vi "myRIO_BRig_RT__Case_Exp_State_Cue1Pre__v3.vi"(0 "input_dataCurrent":u16[](array[numeric]), 1 "input_dataExp":u16[](array[numeric]), 5 "input_arrTrig":bool[](array[boolean]), 6 "input_spout":enum16{"Left", "Right"}(ring)) -> (9 "output_audioR":bool, 11 "output_audioL":bool, 12 "output_state":T1, 13 "output_CueLed":bool, 14 "output_dataCurrent":u16[](array[numeric]), 16 "output_l1_laserEvent":bool, 17 "output_l1_laserOn":bool, 18 "output_l2_laserEvent":bool, 19 "output_l2_laserOn":bool)   [LabVIEW 2014]
uses:
  myRIO_BRig_RT__Case_Exp_stateList.ctl
panel:
  in  "input_I_lick":bool
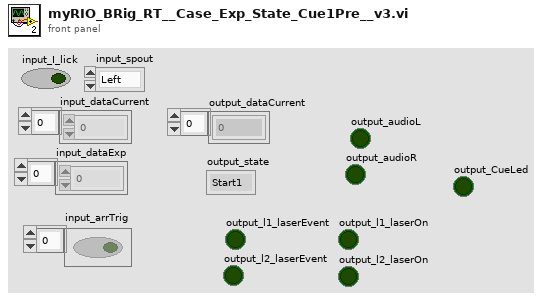
[diagram p1: front panel]
types:
  T1 = typedef "myRIO_BRig_RT__Case_Exp_stateList.ctl" = enum16{"Start1", "Start2", "Start3", "saveSettings1", "saveSettings2", "saveSettings3", "saveSettings4", "saveSettings_LC_ENL_l1", "saveSettings_LC_ENL_l2", "saveSettings_LC_Cue_l1", "saveSettings_LC_Cue_l2", "saveSettings6_LC_l1_Other", "SaveSettings6_LC_l2_Other", "setSettings_Audio", "setSettings_Laser", "initBlock_pre", "initBlock", "initBlock2", "initBlock_post", "initTrial_pre", "initTrial", "initTrial2", "initTrial3", "initTrial4", "initTrial_LC_ENL1", "initTrial_LC_Cue1", "initTrial_LC_Cue1_2", "initTrial_LC_Sel", "initTrial_post", "ENL1_pre", "ENL1", "ENL1_post", "ENL1Penalty_pre", "ENL1Penalty", "ENL2_pre", "ENL2", "ENL2Penalty_pre", "ENL2Penalty", "Cue1_pre", "Cue1", "Cue1_post", "Cue1Penalty_pre", "Cue1Penalty", "Cue2_pre", "Cue2", "Cue2Penalty_pre", "Cue2Penalty", "Selection_pre", "Selection", "Select_post", "SelectReward_pre", "SelectReward", "SelectRewardPost_pre", "SelectRewardPost", "SelectWrong_pre", "SelectWrong", "SelectWrong_post", "SelectTimeout_pre", "SelectTimeout", "SelectTimeout_post", "endTrial_pre", "endTrial1", "endTrial2", "endTrial3", "endTrial_post", "endBlock_pre", "endBlock", "endBlock_post", "endExp", "commConnect", "commUpload_pre", "commUpload_dataBlock", "commUpload_dataCurrent", "commUpload_dataExp", "commUpload_dataLC", "commUpload_dataTrial", "commUpload_post", "saveData_pre", "saveData_dataBlock", "saveData_dataCurrent", "saveData_dataExp", "saveData_dataLC", "saveData_dataTrial", "saveData_post", "empty_endBlock1", "empty_endBlock2", "empty_endTrial1", "empty_endTrial2", "empty_endTrial3", "empty_endTrial4", "empty_endTrial5", "dummyState", "dummyState_endBlock"}
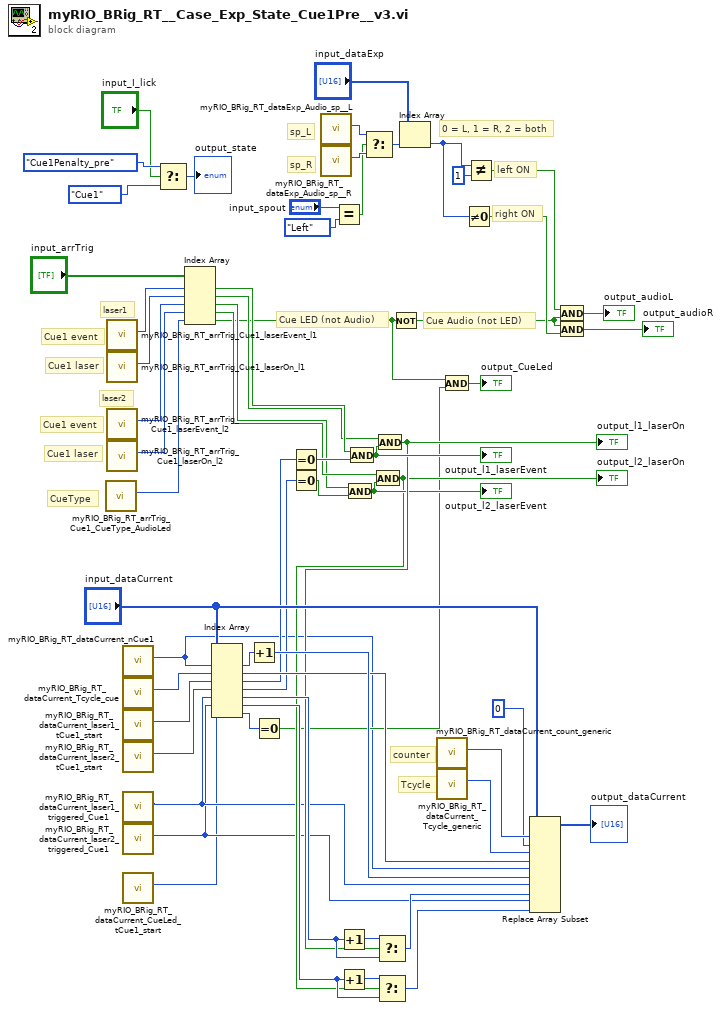
[diagram p0: block diagram]
diagram:
  # "right ON"
  # "left ON"
  # "Cue Audio (not LED)"
  # "Cue LED (not Audio)"
  # "CueType"
  # "0 = L, 1 = R, 2 = both"
  # "sp_R"
  # "sp_L"
  # "Cue1 event"
  # "Cue1 laser"
  # "Cue1 event"
  # "Cue1 laser"
  # "laser2"
  # "laser1"
  # "Tcycle"
  # "counter"
  n1 = call "myRIO_BRig_RT_arrTrig_Cue1_CueType_AudioLed.vi"() -> ("output_arrTrig_Cue1_CueType_AudioLed"=w12:i32)  [unwired: 11 in]
  n2 = call "myRIO_BRig_RT_arrTrig_Cue1_laserEvent_l1.vi"() -> ("output_arrTrig_Cue1_laserEvent_l1"=w25:i32)  [unwired: 11 in]
  n3 = call "myRIO_BRig_RT_arrTrig_Cue1_laserOn_l1.vi"() -> ("output_arrTrig_Cue1_laserOn_l1"=w24:i32)  [unwired: 11 in]
  n4 = call "myRIO_BRig_RT_arrTrig_Cue1_laserEvent_l2.vi"() -> ("output_arrTrig_Cue1_laserEvent_l2"=w23:i32)  [unwired: 11 in]
  n5 = call "myRIO_BRig_RT_arrTrig_Cue1_laserOn_l2.vi"() -> ("output_arrTrig_Cue1_laserOn_l2"=w22:i32)  [unwired: 11 in]
  n6 = call "myRIO_BRig_RT_dataCurrent_nCue1.vi"() -> ("output_nCue1"=w1:i32)  [unwired: 11 in]
  n7 = call "myRIO_BRig_RT_dataCurrent_Tcycle_cue.vi"() -> ("output_Tcycle_cue"=w30:i32)  [unwired: 11 in]
  n8 = call "myRIO_BRig_RT_dataCurrent_laser1_tCue1_start.vi"() -> ("output_laser1_tCue1_start"=w29:i32)  [unwired: 11 in]
  n9 = call "myRIO_BRig_RT_dataCurrent_laser2_tCue1_start.vi"() -> ("output_laser2_tCue1_start"=w28:i32)  [unwired: 11 in]
  n10 = call "myRIO_BRig_RT_dataCurrent_laser1_triggered_Cue1.vi"() -> ("output_laser1_triggered_Cue1"=w27:i32)  [unwired: 11 in]
  n11 = call "myRIO_BRig_RT_dataCurrent_laser2_triggered_Cue1.vi"() -> ("output_laser2_triggered_Cue1"=w26:i32)  [unwired: 11 in]
  n12 = call "myRIO_BRig_RT_dataCurrent_CueLed_tCue1_start.vi"() -> ("output_CueLed_tCue1_start"=w6:i32)  [unwired: 11 in]
  n13 = Select(t=myRIO_BRig_RT__Case_Exp_stateList."Cue1Penalty_pre" ("Enum"), s="input_I_lick", f=myRIO_BRig_RT__Case_Exp_stateList."Cue1" ("Enum")) -> (s? t:f=→"output_state":T1)
  n14 = Index Array(array="input_arrTrig", index #1=w25, index #2=w24, index #3=w23, index #4=w22, index #5=w12) -> (element #1=w40:bool, element #2=w38:bool, element #3=w33:bool, element #4=w34:bool, element #5=w3:bool)
  n15 = Index Array(array="input_dataCurrent", index #1=w1, index #2=w30, index #3=w29, index #4=w28, index #5=w27, index #6=w26, index #7=w6) -> (element #1=w53:u16, element #2=w51:u16, element #3=w50:u16, element #4=w49:u16, element #5=w45:u16, element #6=w44:u16, element #7=w5:u16)
  n16 = Increment(x=w53) -> (x+1=w52:u16)
  n17 = Equal To 0?(x=w5) -> (x = 0?=w4:bool)
  n18 = Equal To 0?(x=w50) -> (x = 0?=w41:bool)
  n19 = Equal To 0?(x=w49) -> (x = 0?=w32:bool)
  n20 = call "myRIO_BRig_RT_dataExp_Audio_sp__L.vi"() -> ("output_Audio_sp__L"=w17:i32)  [unwired: 11 in]
  n21 = call "myRIO_BRig_RT_dataExp_Audio_sp__R.vi"() -> ("output_Audio_sp__R"=w18:i32)  [unwired: 11 in]
  n22 = Equal?(x="input_spout", y=enum16{"Left", "Right"}."Left") -> (x = y?=w16:bool)
  n23 = Increment(x=w45) -> (x+1=w47:u16)
  n24 = Increment(x=w44) -> (x+1=w46:u16)
  n25 = And(x=w33, y=w32) -> (x .and. y?=w36:bool)
  "output_l2_laserEvent" <- w36
  n26 = And(x=w40, y=w41) -> (x .and. y?=w39:bool)
  "output_l1_laserEvent" <- w39
  n27 = Select(t=w17, s=w16, f=w18) -> (s? t:f=w19:i32)
  n28 = And(x=w34, y=w36) -> (x .and. y?=w35:bool)
  "output_l2_laserOn" <- w35
  n29 = And(x=w38, y=w39) -> (x .and. y?=w37:bool)
  "output_l1_laserOn" <- w37
  n30 = Select(t=w47, s=w37, f=w45) -> (s? t:f=w43:u16)
  n31 = Select(t=w46, s=w35, f=w44) -> (s? t:f=w42:u16)
  n32 = Not(x=w3) -> (.not. x?=w9:bool)
  n33 = Index Array(array="input_dataExp", index=w19) -> (element=w21:u16)
  n34 = call "myRIO_BRig_RT_dataCurrent_count_generic.vi"() -> ("output_count_generic"=w56:i32)  [unwired: 11 in]
  n35 = call "myRIO_BRig_RT_dataCurrent_Tcycle_generic.vi"() -> ("output_Tcycle_generic"=w55:i32)  [unwired: 11 in]
  n36 = And(x=w3, y=w4) -> (x .and. y?=→"output_CueLed":bool)
  n37 = Not Equal To 0?(x=w21) -> (x != 0?=w10:bool)
  n38 = Not Equal?(x=w21, y=u16 1) -> (x != y?=w11:bool)
  n39 = Replace Array Subset(array="input_dataCurrent", new element #1=u16 0 ("new element/subarray"), index #1=w56, new element #2=w51, index #2=w55, new element #3=w52, index #3=w1, new element #4=w43, index #4=w27, new element #5=w42, index #5=w26) -> (→"output_dataCurrent":u16[])
  n40 = And(x=w11, y=w9) -> (x .and. y?=→"output_audioL":bool)
  n41 = And(x=w9, y=w10) -> (x .and. y?=→"output_audioR":bool)
